vi "InitPic.vi"(2 "Cluster of 7 Type Data":T2(array[cluster])) -> (1 "Image Out 2":T3)   [LabVIEW 2014]
doc: "转换二维图片为像素图"
uses:
  <vilib>/vision/Image Controls.llb/IMAQ Image.ctl
  <vilib>/Analysis/Matrix/Datatypes/RealMatrix.ctl
  <vilib>/Analysis/Matrix/NI_Matrix.lvlib
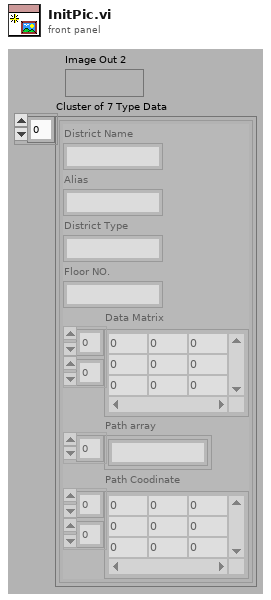
[diagram p1: front panel]
types:
  T1 = typedef "NI_Matrix.lvlib/RealMatrix.ctl" = dbl[][]
  T2 = cluster{"District Name":string, "Alias":string, "District Type":string, "Floor NO.":string, "Data Matrix":T1, "Path array":string[], "Path Coodinate":T1}[]
  T3 = typedef "IMAQ Image.ctl" = refnum<image>
  T4 = typedef "imagedata.ctl" = cluster{"image type":i32, "image depth":i32, "image":u8[], "mask":u8[], "colors":u32[], "Rectangle":cluster{"left":i16, "top":i16, "right":i16, "bottom":i16}}
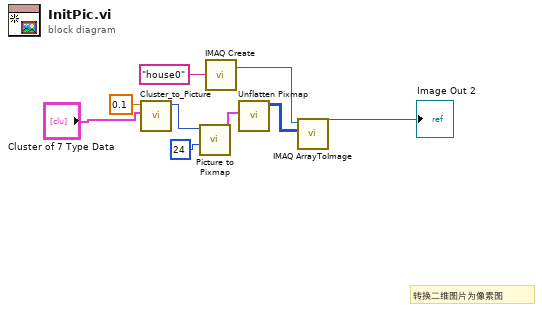
[diagram p0: block diagram]
diagram:
  # "转换二维图片为像素图"
  n1 = call "Cluster_to_Picture.vi"("Cluster of 7 Type Data"="Cluster of 7 Type Data", "Scalar"=0.1) -> ("Anto Drawer"=w2:picture)  [unwired: 9 in]
  n2 = call <vilib>:"Picture to Pixmap.vi"("depth"=24, "picture"=w2) -> ("image data"=w7:T4)  [unwired: 8 in, 1 out]
  n3 = call "IMAQ Create"("Image Name"="house0") -> ("New Image"=w6:T3)  [unwired: 4 in, 1 out]
  n4 = call <vilib>:"Unflatten Pixmap.vi"("image data"=w7) -> ("24-bit pixmap"=w8:u32[][])  [unwired: 4 in, 6 out]
  n5 = call "IMAQ ArrayToImage"("Image Pixels (U8)"=w8, "Image"=w6) -> ("Image Out"=→"Image Out 2":T3)  [unwired: 8 in, 1 out]
